vi "Get Number of Channels.vi"(4 "Channel":string[](array[string])=["[globals]", "project", "partnumber", "setup_image", "[channel_1]", "mode", "dmm_mode", "ps-source_mode", "switch_settings", "comment", "[channel_2]"]) -> (1 "# Channels":i32)   [LabVIEW 2015]
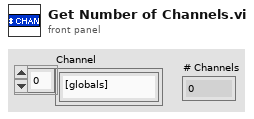
[diagram p1: front panel]
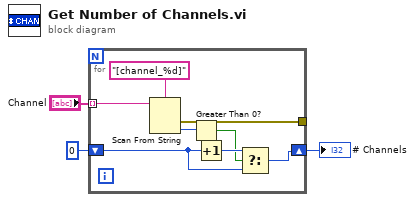
[diagram p0: block diagram]
diagram:
  n1 = for {
    tunnel: "Channel" -> [w11] mode=indexing
    shift-right: [w6] -> w1
    shift-left: 0 -> [w7]
    tunnel: [w4] -> _
    n2 = Scan From String(format string="[channel_%d]", input string=w11) -> (error out=w4:errorcluster, output 1=w9:i32)  [unwired: 3 in, 2 out]
    n3 = Greater Than 0?(x=w9) -> (x > 0?=w5:bool)
    n4 = Increment(x=w7) -> (x+1=w8:i32)
    n5 = Select(t=w8, s=w5, f=w7) -> (s? t:f=w6:i32)
  }
  "# Channels" <- w1
